vi "Three Session Two Pins Three Instrument Two Sites - DMM.vi"(8 "error in":errorcluster) -> (0 "error out":errorcluster, 3 "session reservation out":refnum<class "Session Reservation.lvclass">)   [LabVIEW 2020, in "MeasurementServerTests.lvlib"]
uses:
  MeasurementServerTests.lvlib
  TestUtilities/TestUtilities.Runtime/Session Reservation Test Utilities/Session Reservation Test Utilities.lvlib
  Runtime/Measurements/Measurement Plugin Session Management V1/Session Reservation/Session Reservation.lvclass
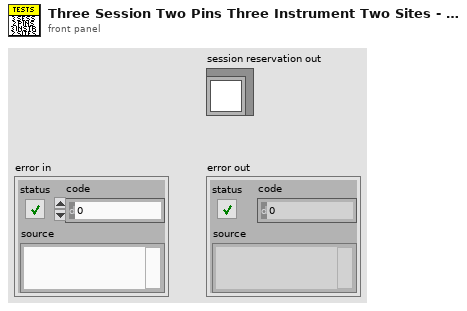
[diagram p1: front panel]
types:
  T1 = typedef "Measurement Plugin Session Management V1.lvlib/Session Reservation.lvclass/Data.ctl" = cluster{"session and driver infos":T2[], "pin or relay names":string[], "connection map":refnum<class "Connection Map.lvclass">, "pin map context":T7, "reservation observer":refnum<class "IReservation Observer.lvclass">, "dvr valid":bool, "group mappings":T8}
  T2 = typedef "Measurement Plugin Session Management V1.lvlib/Session Reservation.lvclass/Session and Driver Info.ctl" = cluster{"session info":T3, "session":variant, "session factory":refnum<class "ISession Factory.lvclass">, "initialize and close session behavior":T6}
  T3 = typedef "MeasurementLink Session Management Client.lvlib/ni_measurementlink_sessionmanagement_v1_SessionInformation.ctl" = cluster{"session":T4, "resource_name":string, "channel_list":string, "instrument_type_id":string, "session_exists":bool, "channel_mappings":T5[]}
  T4 = typedef "MeasurementLink Session Management Client.lvlib/nidevice_grpc_Session.ctl" = cluster{"name":string}
  T5 = typedef "MeasurementLink Session Management Client.lvlib/ni_measurementlink_sessionmanagement_v1_ChannelMapping.ctl" = cluster{"pin_or_relay_name":string, "site":i32, "channel":string, "multiplexer_resource_name":string, "multiplexer_route":string}
  T6 = typedef "MeasurementLink Instrument.lvlib/ISession Factory.lvclass/Initialize and Close Session Behavior.ctl" = enum16{"Initialize and Close", "Attach and Detach", "Initialize and Detach", "Attach and Close"}
  T7 = typedef "MeasurementLink Session Management Client.lvlib/ni_measurementlink_PinMapContext.ctl" = cluster{"pin_map_id":string, "sites":i32[]}
  T8 = typedef "Measurement Plugin Session Management V1.lvlib/Session Reservation.lvclass/Group Mapping.ctl" = map{string, string[]}
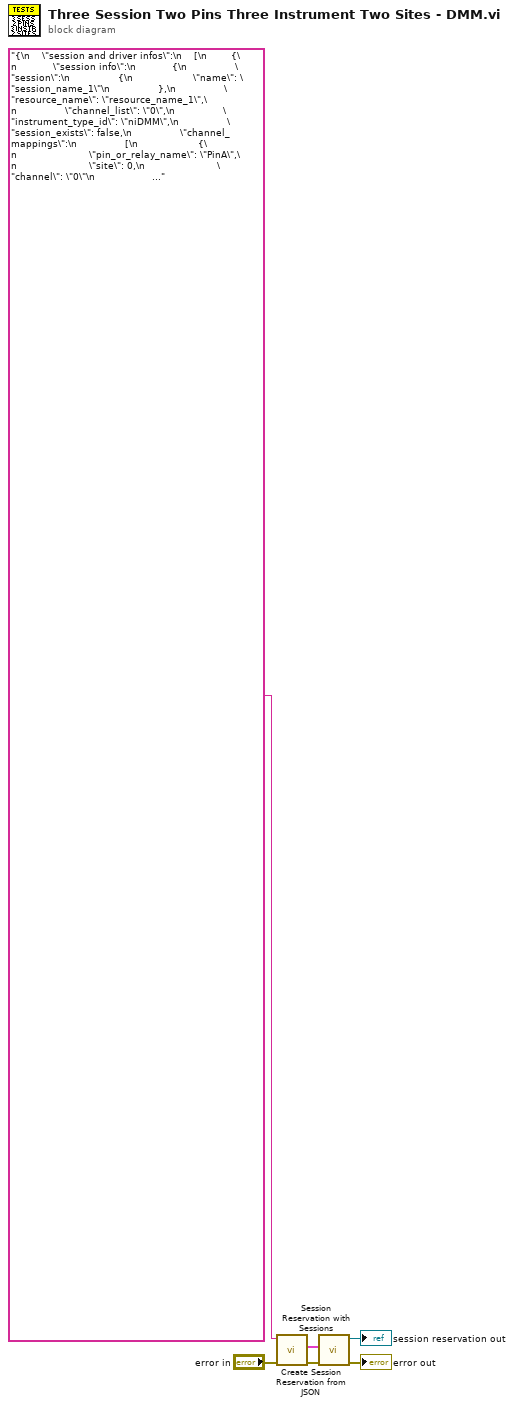
[diagram p0: block diagram]
diagram:
  n1 = call "Create Session Reservation from JSON.vi"("error in"="error in", "json"="{\n    \"session and driver infos\":\n    [\n        {\n            \"session info\":\n            {\n                \"session\":\n                {\n                    \"name\": \"session_name_1\"\n                },\n                \"resource_name\": \"resource_name_1\",\n                \"channel_list\": \"0\",\n                \"instrument_type_id\": \"niDMM\",\n                \"session_exists\": false,\n                \"channel_mappings\":\n                [\n                    {\n                        \"pin_or_relay_name\": \"PinA\",\n                        \"site\": 0,\n                        \"channel\": \"0\"\n                    },\n                ]\n            },\n            \"session\": \"\"\n        },\n        {\n\t\t\t\"session info\":\n            {\n                \"session\":\n                {\n                    \"name\": \"session_name_2\"\n                },\n                \"resource_name\": \"resource_name_2\",\n                \"channel_list\": \"0\",\n                \"instrument_type_id\": \"niDMM\",\n                \"session_exists\": false,\n                \"channel_mappings\":\n                [\n                    {\n                        \"pin_or_relay_name\": \"PinB\",\n                        \"site\": 0,\n                        \"channel\": \"0\"\n                    },\n                ]\n            },\n            \"session\": \"\"\n        },\n\t\t{\n\t\t\t\"session info\":\n            {\n                \"session\":\n                {\n                    \"name\": \"session_name_3\"\n                },\n                \"resource_name\": \"resource_name_3\",\n                \"channel_list\": \"0\",\n                \"instrument_type_id\": \"niDMM\",\n                \"session_exists\": false,\n                \"channel_mappings\":\n                [\n                    {\n                        \"pin_or_relay_name\": \"PinA\",\n                        \"site\": 1,\n                        \"channel\": \"0\"\n                    },\n                ]\n            },\n            \"session\": \"\"\n        }\n    ],\n    \"pin or relay names\":\n    [\n        \"PinA\",\n        \"PinB\"\n    ],\n    \"pin map context\":\n    {\n        \"pin_map_id\": \"pin_map_id_1\",\n        \"sites\":\n        [\n            0,\n            1\n        ]\n    },\n    \"dvr valid\": true\n}") -> ("error out"=w6:errorcluster, "data out"=w5:T1)  [unwired: 7 in, 1 out]
  n2 = call "Session Reservation with Sessions.vi"("error in"=w6, "data in"=w5) -> ("error out"=→"error out":errorcluster, "session reservation out"=→"session reservation out":refnum<class "Session Reservation.lvclass">)  [unwired: 7 in, 1 out]
